vi "EPICS Time Stamp to Time Stamp.vi"(0 "EPICS time stamp":T1) -> (1 "user tag":i32, 2 "time stamp":timestamp)   [LabVIEW 2020, in "PV Access.lvlib" / "PV Data.lvlib"]
uses:
  PV Data.lvlib
  EPICS Time Stamp.ctl
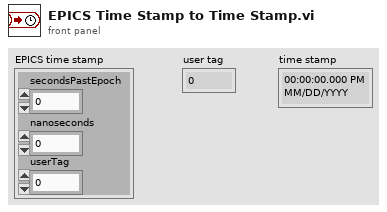
[diagram p1: front panel]
types:
  T1 = typedef "PV Access.lvlib/PV Data.lvlib/EPICS Time Stamp.ctl" = cluster{"secondsPastEpoch":i64, "nanoseconds":i32, "userTag":i32}
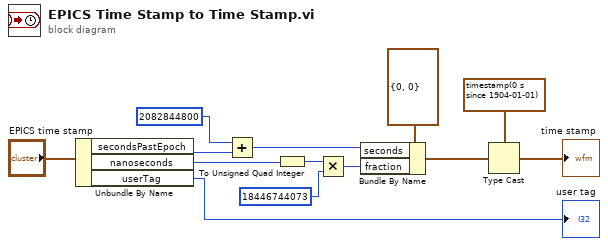
[diagram p0: block diagram]
diagram:
  n1 = Unbundle By Name("EPICS time stamp") -> ("secondsPastEpoch"=w8:i64, "nanoseconds"=w5:i32, "userTag"=→"user tag":i32)
  n2 = Add(x=i64 2082844800 ("y"), y=w8) -> (x+y=w6:i64)
  n3 = To Unsigned Quad Integer(1:w5) -> (0:w4:u64)
  n4 = Multiply(x=w4, y=u64 18446744073) -> (x*y=w2:u64)
  n5 = Bundle By Name(cluster=cluster{"seconds":i64, "fraction":u64} {"seconds"=0, "fraction"=0}, "seconds"=w6, "fraction"=w2) -> (w11:cluster{"seconds":i64, "fraction":u64})
  n6 = Type Cast(type=timestamp(0 s since 1904-01-01), x=w11) -> (*(type *) &x=→"time stamp":timestamp)
